vi "YawOverflows.vi"(1 "Yaw (degrees)":dbl) -> (0 "Yaw (with overflows)":dbl)   [LabVIEW 2014, in "Team900SwerveDrive.lvlib"]
uses:
  Team900SwerveDrive.lvlib
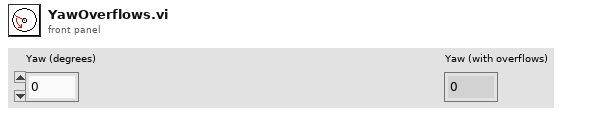
[diagram p1: front panel]
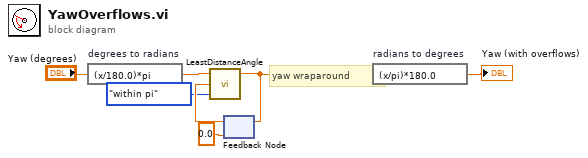
[diagram p0: block diagram]
diagram:
  # "yaw wraparound"
  n1 = expression code="(x/180.0)*pi" "degrees to radians"("Yaw (degrees)") -> (w3:dbl)
  n2 = feedback #1(0.0) -> (w4:dbl)
  n3 = call "LeastDistanceAngle.vi"("Enum"=enum16{"within pi", "within pi/2"}."within pi", "Current angle"=w4, "target angle (between pi and -pi) 2"=w3) -> ("output angle"=w1:dbl)  [unwired: 2 out]
  n4 = feedback-in #1(w1) -> ()
  n5 = expression code="(x/pi)*180.0" "radians to degrees"(w1) -> (→"Yaw (with overflows)":dbl)
